vi "PieChart-Properties.vi"(5 "Yeild-chart 2":refnum<vi>, 6 "Plot Cluster Index out":cluster{"Plot Cluster":T1, i32}, 7 "Label Total":refnum<vi>, 8 "error in (no error)":errorcluster, 9 "Zen Analytics in":refnum<class "Zen Analytics.lvclass">, 10 "Lable":picture, 11 "YeildChart":picture) -> (0 "error out":errorcluster)   [LabVIEW 2019, in "Zen Analytics.lvlib" / "Zen Analytics.lvclass"]
uses:
  Zen Analytics.lvclass
  Dependency/GraphReff.ctl
  <vilib>/ActorFramework/Message Enqueuer/Message Enqueuer.lvclass
  Dependency/AnalyticsDataToSM.ctl
  Dependency/Plot Cluster.ctl
types:
  T1 = typedef "Zen Analytics.lvlib/Zen Analytics.lvclass/Plot Cluster.ctl" = cluster{"Reduced 2D":dbl[][], "Start Index":i32, "No Of New Termnals":i32, "Top/Bottom":bool, "Values Inserted":i32, "Re-Initialised":bool, "Statistical params":string[][], "MeasurementInitializationData":cluster{"Measurement-ID":i32[], "Measurement Names":string[], "NominalValues":dbl[], "LSL":dbl[], "USL":dbl[], "LCL":dbl[], "UCL":dbl[]}, "MeasurementData":cluster{"Measurement ID":i32, "Measurement Name":string, "Nominal Values":dbl, "LSL":dbl, "USL":dbl, "LCL":dbl, "UCL":dbl}[], "ResultData2D":dbl[][], "PlotParameters":cluster{"Trend":cluster{"TrendPlotID":dbl, "PlotProperties":cluster{"FontName":string, "FontSize":dbl, "FontColor":string, "IsBold":bool, "IsItalic":bool, "PlotColor":string}}[], "Histogram":cluster{"HistogramPlotID":dbl, "PlotProperties":cluster{"FontName":string, "FontSize":dbl, "FontColor":string, "IsBold":bool, "IsItalic":bool, "PlotColor":string}}[], "BarPlot":cluster{"BarPlotID":dbl, "BarValuesID":dbl, "PlotProperties":cluster{"FontName":string, "FontSize":dbl, "IsBold":bool, "IsItalic":bool, "FontColor":string}, "Sectors":string[]}[], "PieChart":cluster{"PieChartID":dbl, "PieChartValueID":dbl, "PlotProperties":cluster{"FontName":string, "FontSize":dbl, "IsBold":bool, "IsItalic":bool, "FontColor":string}, "Sectors":string[]}[]}}
  T2 = cluster{"PieChartID":dbl, "PieChartValueID":dbl, "PlotProperties":cluster{"FontName":string, "FontSize":dbl, "IsBold":bool, "IsItalic":bool, "FontColor":string}, "Sectors":string[]}[]
  T3 = cluster{"PieChartID":dbl, "PieChartValueID":dbl, "PlotProperties":cluster{"FontName":string, "FontSize":dbl, "IsBold":bool, "IsItalic":bool, "FontColor":string}, "Sectors":string[]}
  T4 = typedef "Zen Analytics.lvlib/Zen Analytics.lvclass/AnalyticsDataToSM.ctl" = cluster{"Actor Info":cluster{"Analytics Enqueuer":refnum<class "Message Enqueuer.lvclass">, "This VI":refnum<vi>, "Module name":string}, "Statistical Info":string[][], "Graph Refference's":T5, "ErrorMessage":string}
  T5 = typedef "Zen Analytics.lvlib/Zen Analytics.lvclass/GraphReff.ctl" = cluster{"HistgramGraph-reff":refnum<vi>[], "BarGraph-reff":refnum<vi>[], "PieGraph-reff":refnum<vi>[], "Lable-reff":refnum<vi>[], "TrendGraph-reff":refnum<vi>[], "CpCpkTable":refnum<vi>}
  T6 = cluster{"FontName":string, "FontSize":dbl, "IsBold":bool, "IsItalic":bool, "FontColor":string}
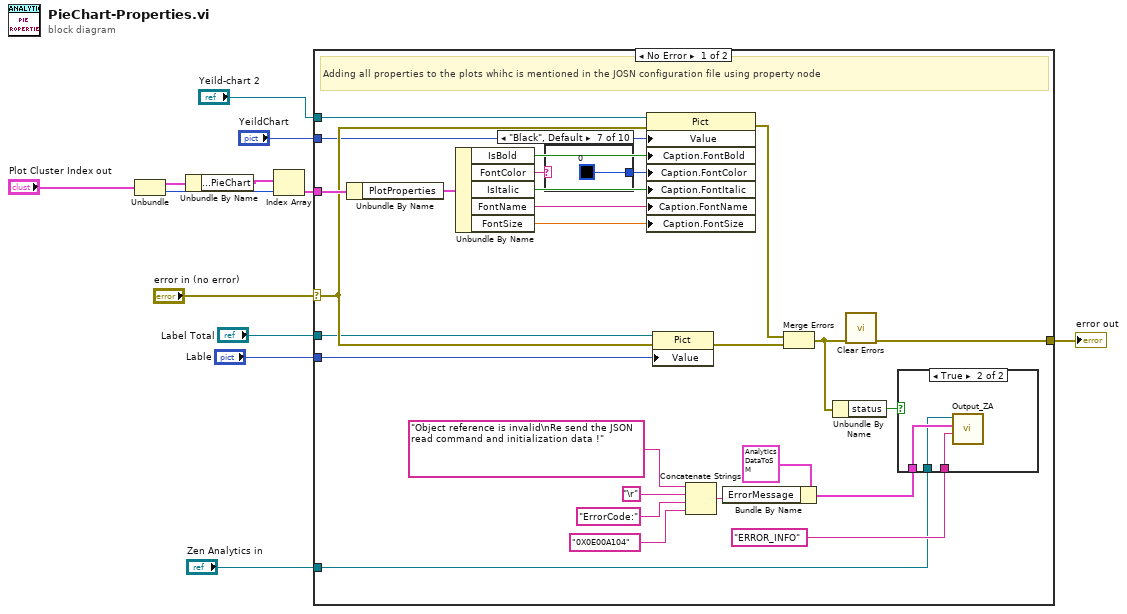
[diagram p0: block diagram]
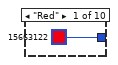
[diagram p3: hidden frame]
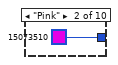
[diagram p4: hidden frame]
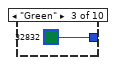
[diagram p5: hidden frame]
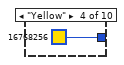
[diagram p6: hidden frame]
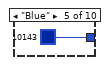
[diagram p7: hidden frame]
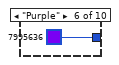
[diagram p8: hidden frame]
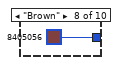
[diagram p9: hidden frame]
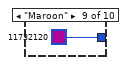
[diagram p10: hidden frame]
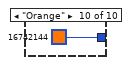
[diagram p11: hidden frame]
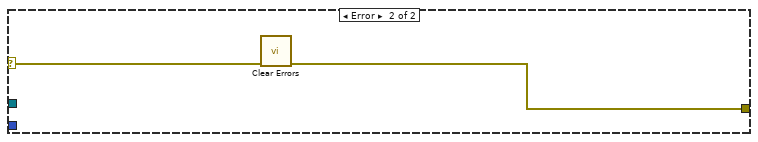
[diagram p12: hidden frame]
diagram:
  n1 = Unbundle("Plot Cluster Index out") -> ("Plot Cluster"=w5:T1, w7:i32)
  n2 = Unbundle By Name(w5) -> ("PlotParameters.PieChart"=w4:T2)
  n3 = Index Array(array=w4, index=w7) -> (element=w3:T3)
  n4 = case shown="No Error" "error in (no error)" {
    selector: "error in (no error)" -> [w37 w54]
    tunnel: w3 -> [w39 _]
    tunnel: "YeildChart" -> [w26 _]
    tunnel: "Yeild-chart 2" -> [w38 _]
    tunnel: [w16 w53] -> w2
    tunnel: "Lable" -> [w36 _]
    tunnel: "Label Total" -> [w35 _]
    tunnel: "Zen Analytics in" -> [w13 _]
    frame No Error {
      # "Adding all properties to the plots whihc is mentioned in the JOSN configuration file using property node"
      n5 = Unbundle By Name(w39) -> ("PlotProperties"=w34:T6)
      n6 = Unbundle By Name(w34) -> ("IsBold"=w30:bool, "FontColor"=w29:string, "IsItalic"=w31:bool, "FontName"=w32:string, "FontSize"=w33:dbl)
      n7 = case shown="\"Black\", Default" w29 {
        tunnel: [u32 15663122 u32 15073510 u32 32832 u32 16768256 u32 10143 u32 7995636 u32 0 u32 8405056 u32 11732120 u32 16742144] -> w28
        frame "Red" {
        }
        frame "Pink" {
        }
        frame "Green" {
        }
        frame "Yellow" {
        }
        frame "Blue" {
        }
        frame "Purple" {
        }
        frame "Black", Default {
        }
        frame "Brown" {
        }
        frame "Maroon" {
        }
        frame "Orange" {
        }
      }
      n8 = property on="Property Node" class="Pict"(reference=w38, error in=w37, "Value"=w26, "Caption.FontBold"=w30, "Caption.FontColor"=w28, "Caption.FontItalic"=w31, "Caption.FontName"=w32, "Caption.FontSize"=w33) -> (error out=w27:errorcluster)  [unwired: 1 out]
      n9 = property on="Property Node" class="Pict"(reference=w35, error in=w37, "Value"=w36) -> (error out=w25:errorcluster)  [unwired: 1 out]
      n10 = Concatenate Strings("Object reference is invalid\nRe send the JSON read command and initialization data !" ("SolutionForError"), "\r", "ErrorCode:", "0X0E00A104" ("ErrorCode")) -> (w19:string)
      n11 = Bundle By Name(cluster=T4 {"Actor Info"={"Analytics Enqueuer"=refnum, "This VI"=refnum, "Module name"=""}, "Statistical Info"=[], "Graph Refference's"={"HistgramGraph-reff"=[], "BarGraph-reff"=[], "PieGraph-reff"=[], "Lable-reff"=[], "TrendGraph-reff"=[], "CpCpkTable"=refnum}, "ErrorMessage"=""} ("Analytics Information"), "ErrorMessage"=w19) -> (w18:T4)
      n12 = Merge Errors(w27, w25) -> (w15:errorcluster)
      n13 = Unbundle By Name(w15) -> ("status"=w14:bool)
      n14 = call <vilib>:"Clear Errors.vi"("error in (no error)"=w15) -> ("error out"=w16:errorcluster)  [unwired: 5 in, 1 out]
      n15 = case shown="True" w14 {
        tunnel: w18 -> [_ w42]
        tunnel: "ERROR_INFO" ("State") -> [_ w41]
        tunnel: w13 -> [_ w40]
        frame False {
        }
        frame True {
          n16 = call "Output_ZA.vi"("State"=w41, "Analytics Information"=w42, "Zen Analytics in"=w40) -> ()  [unwired: 7 in, 2 out]
        }
      }
    }
    frame Error {
      n17 = call <vilib>:"Clear Errors.vi"("error in (no error)"=w54) -> ("error out"=w53:errorcluster)  [unwired: 5 in, 1 out]
    }
  }
  "error out" <- w2
